vi "UI_GUI.vi"() -> ()   [LabVIEW 2014]
uses:
  <vilib>/addons/database/Connection.llb/DB Tools Open Connec (String).vi
  <vilib>/Utility/file.llb/Read From Spreadsheet File (string).vi
  Terminal-Global-SetValues.vi
  <vilib>/addons/database/_DB Variant To Data/Database Variant To Data.xnode
  <vilib>/addons/database/NI_Database_API.lvlib
panel:
  in  "取消":bool
  in  "选项卡控件":enum32{"选项卡 1", "选项卡 2", "选项卡 3", "选项卡 4"}(tab)
  in  "NEXT_1":bool caption="下一步"
  in  "试验人员姓名":string
  in  "试验名称":string
  out "试验日期":string
  in  "径向加载压力":dbl
  in  "轴向加载压力":dbl
  in  "润滑油温度":dbl
  in  "轴承类型":enum32{"角接触球", "圆柱滚子"}(radio)
  in  "BACK_2":bool caption="上一步"
  in  "NEXT_2":bool caption="下一步"
  in  "供油流量":dbl
  in  "供油润滑油温度":dbl caption="供油润滑油温度T"
  in  "下拉列表":u16(ring) items=["", "模板一", "模板二", "模板三"]
  in  "选择文件":path
  in  "BACK_3":bool caption="上一步"
  in  "NEXT_3":bool caption="下一步"
  in  "载荷谱表格":string[][](table)
  out "载荷谱表格显示":string[][](table) caption="载荷谱表格"
  out "润滑油温度显示":dbl caption="润滑油温度"
  out "轴承类型显示":string caption="轴承类型"
  in  "BACK_4":bool caption="上一步"
  out "试验日期显示":string caption="试验日期"
  out "试验人员姓名显示":string caption="试验人员姓名"
  out "试验名称显示":string caption="试验名称"
  out "径向加载压力显示":dbl caption="径向加载压力"
  out "轴向加载压力显示":dbl caption="轴向加载压力"
  out "供油润滑油温度显示":dbl caption="供油润滑油温度T"
  out "供油流量显示":dbl caption="供油流量"
  in  "ok":bool
  # "轴承测试系统"
  # "试验信息输入"
  # "试验轴承类型"
  # "请选择"
  # "试验轴承润滑单元设定"
  # "预载荷及高压顶起载荷设置"
  # "载荷谱设置"
  # "选择载荷谱模板"
  # "导入载荷谱"
  # "请确认您输入的内容"
  # "试验轴承润滑单元参数"
  # "预载荷及高压顶起载荷设置"
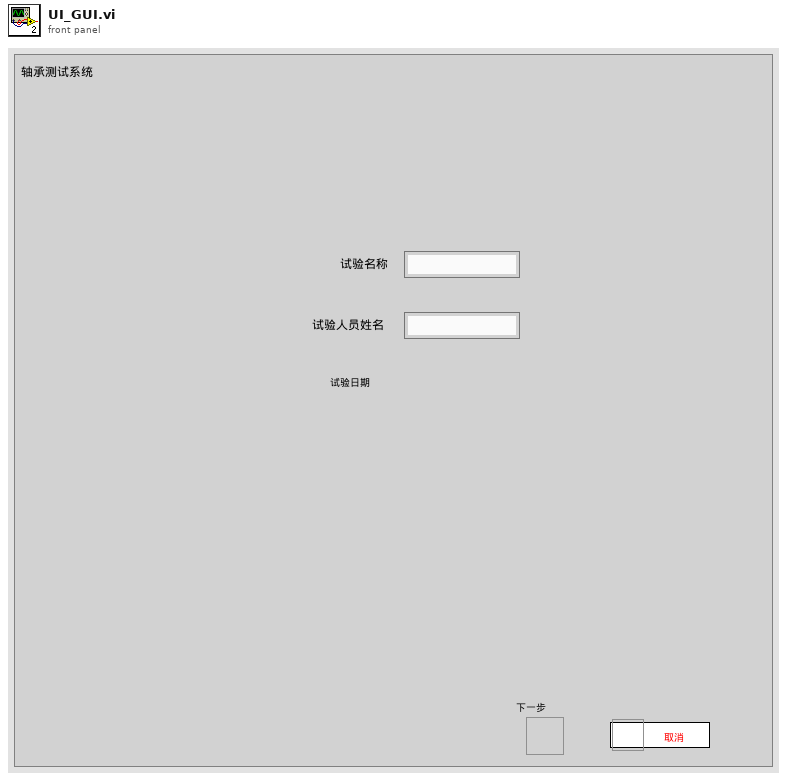
[diagram p1: front panel]
types:
  T1 = enum32{"选项卡 1", "选项卡 2", "选项卡 3", "选项卡 4", "选项卡 5", "选项卡 6", "选项卡 7"}
  T2 = typedef "NI_Database_API.lvlib/Conn ObjectReference.ctl" = refnum<k1>
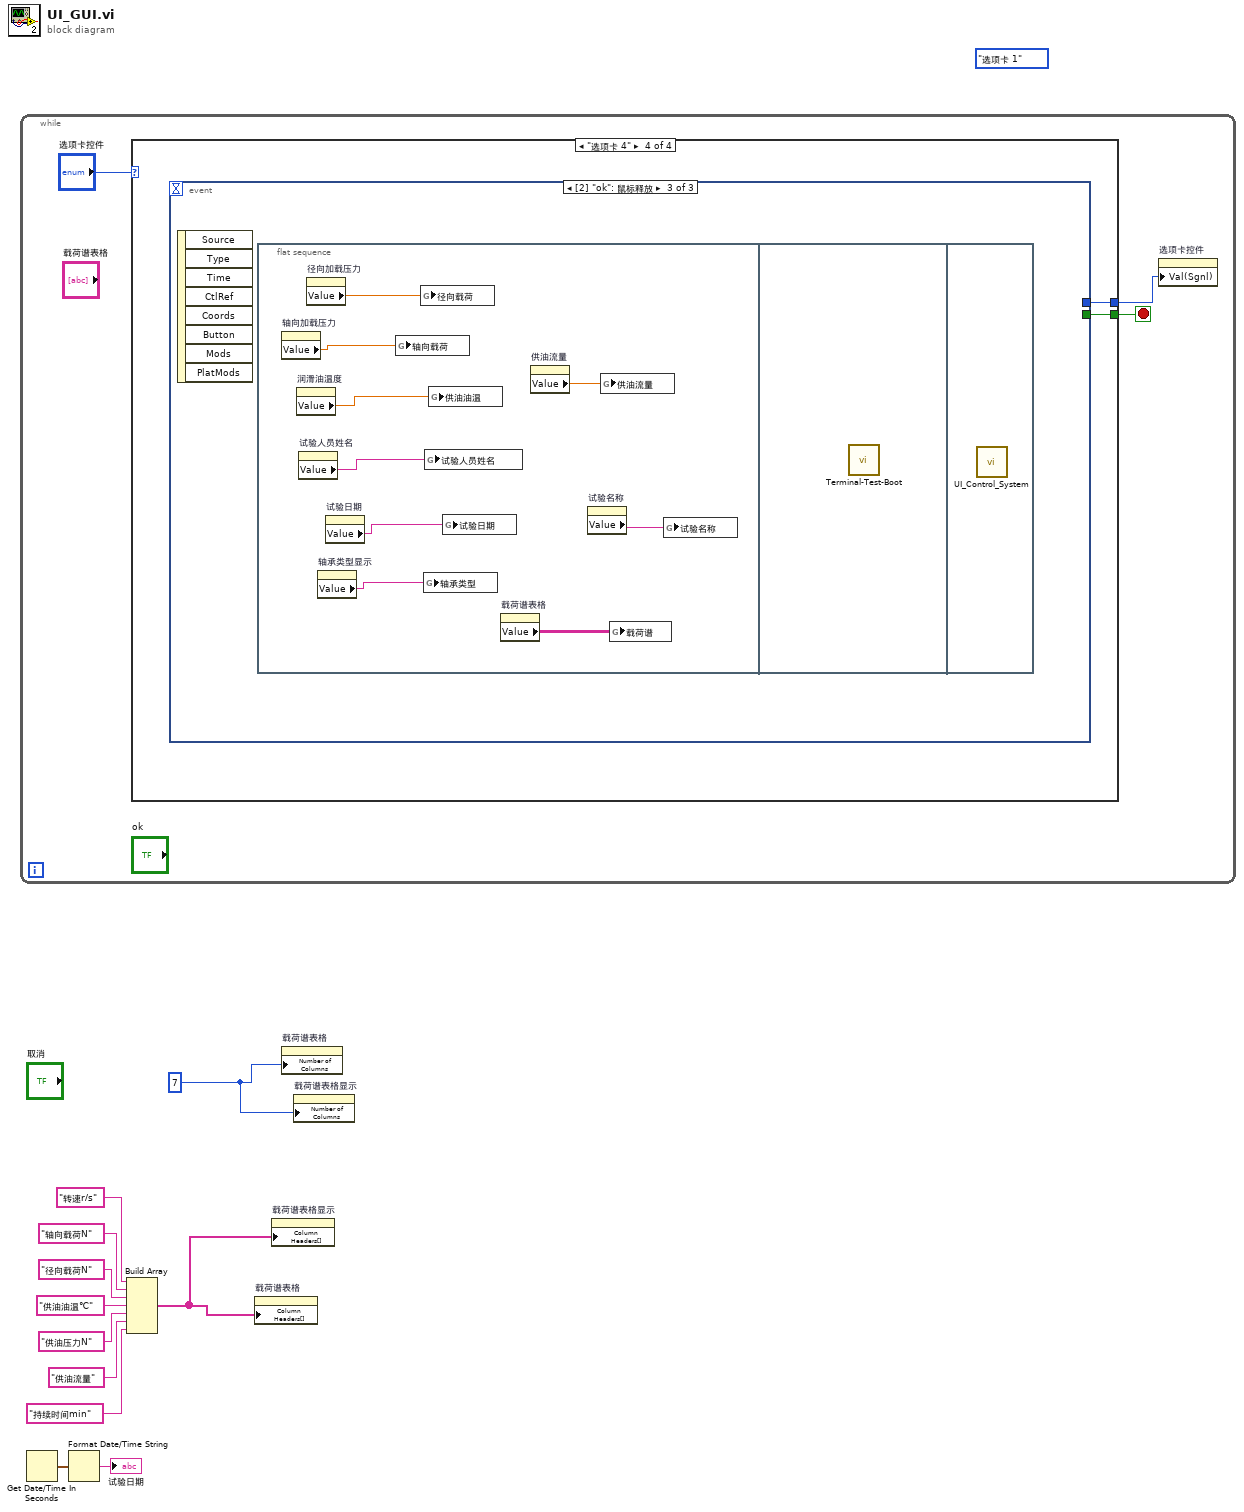
[diagram p0: block diagram]
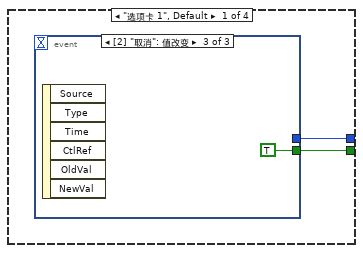
[diagram p2: hidden frame]
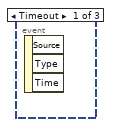
[diagram p3: hidden frame]
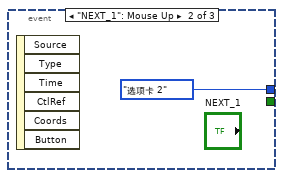
[diagram p4: hidden frame]
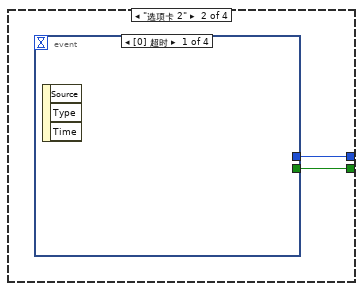
[diagram p5: hidden frame]
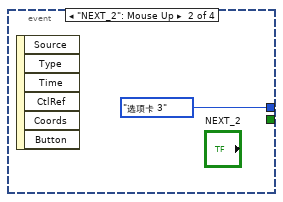
[diagram p6: hidden frame]
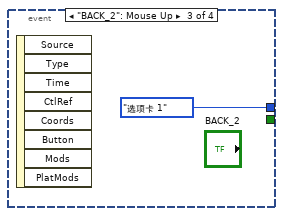
[diagram p7: hidden frame]
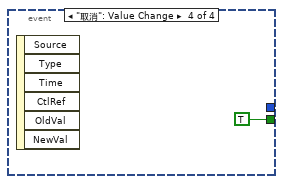
[diagram p8: hidden frame]
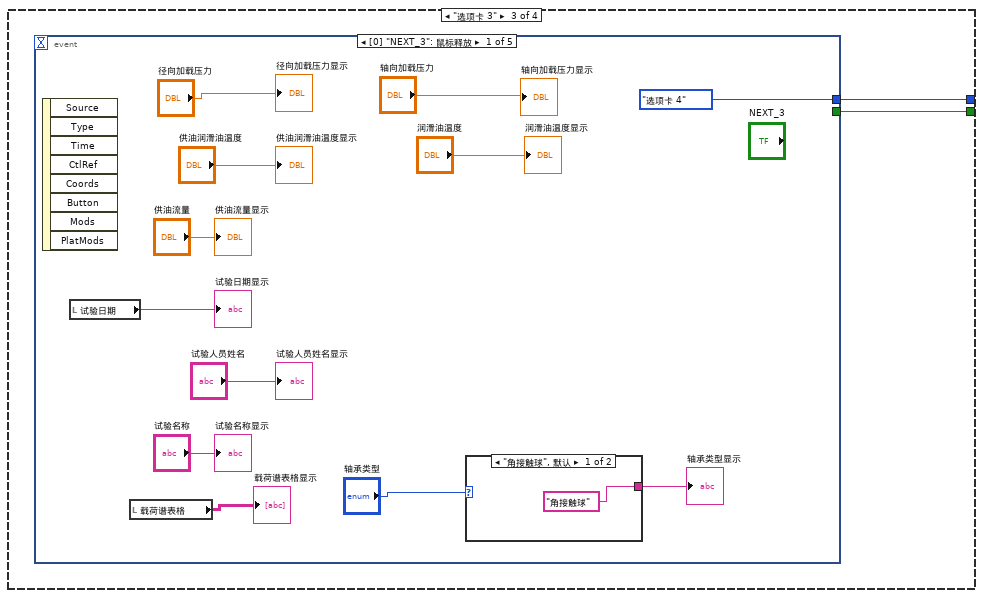
[diagram p9: hidden frame]
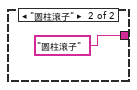
[diagram p10: hidden frame]
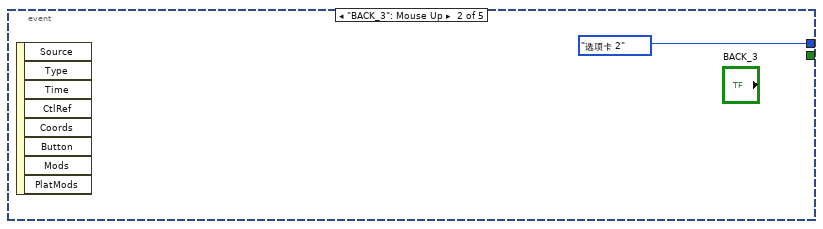
[diagram p11: hidden frame]
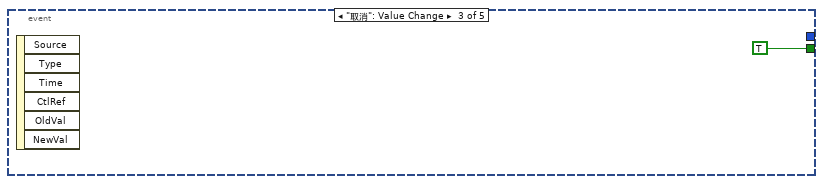
[diagram p12: hidden frame]
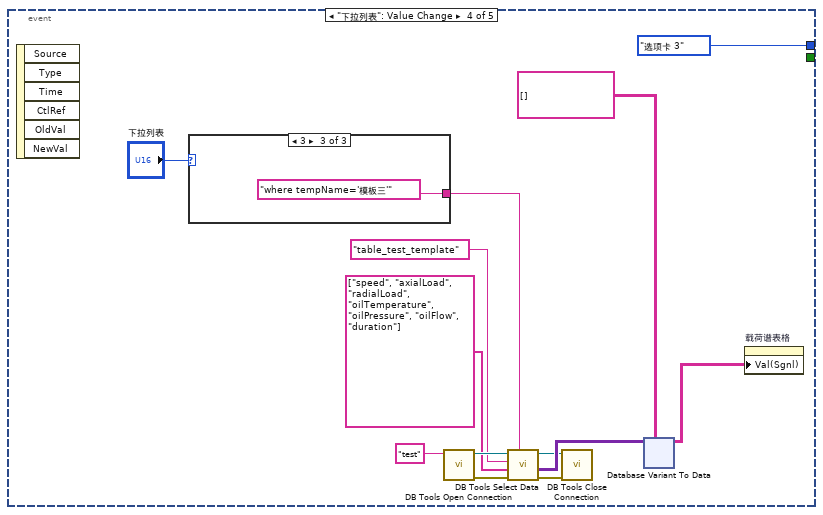
[diagram p13: hidden frame]
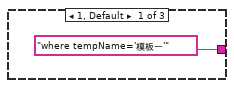
[diagram p14: hidden frame]
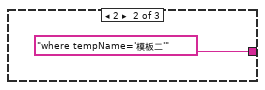
[diagram p15: hidden frame]
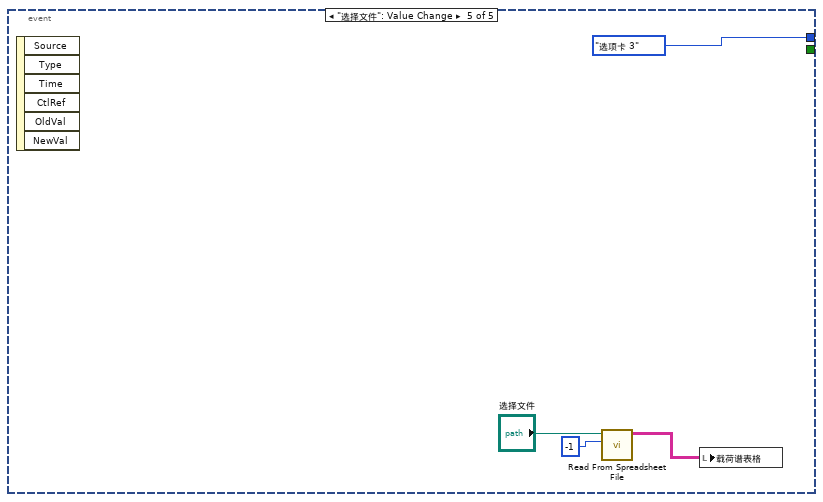
[diagram p16: hidden frame]
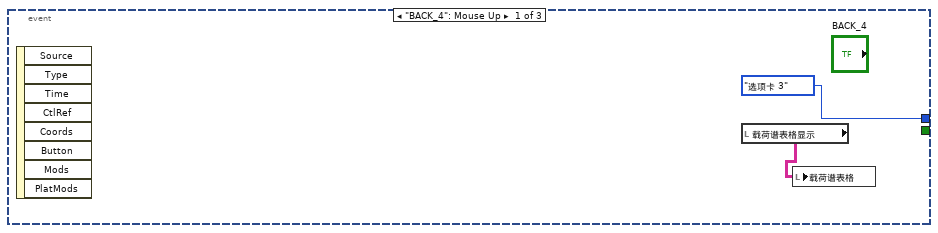
[diagram p17: hidden frame]
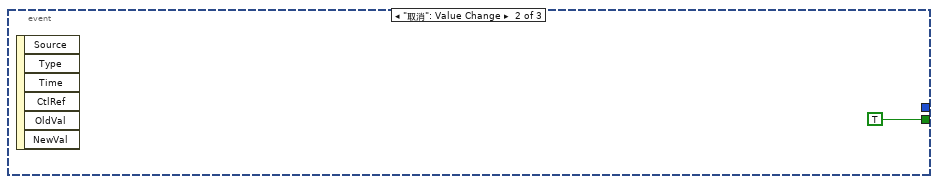
[diagram p18: hidden frame]
diagram:
  w1 = 7
  (unwired) enum32{"选项卡 1", "选项卡 2", "选项卡 3", "选项卡 4"}."选项卡 1" ("选项卡控件")
  n1 = while {
    stop <- w13 stop-if-true
    n2 = case shown="\"选项卡 4\"" "选项卡控件" {
      tunnel: [w16 w20 w25 w107] -> w14
      tunnel: [w15 w19 w24 w106] -> w13
      frame "选项卡 1", Default {
        n3 = event shown="[2] \"取消\": 值改变" {
          selector: _ -> [_ _ _]
          dyn-events: _ -> [_ _ _]
          timeout: _ -> [_ _ _]
          tunnel: [_ T1."选项卡 2" ("选项卡控件") _] -> w16
          tunnel: [_ _ TRUE] -> w15
          event Timeout {
            n4 = event-data() -> ()  [unwired: 1 in, 3 out]
          }
          event "NEXT_1": Mouse Up {
            n5 = event-data() -> ()  [unwired: 1 in, 6 out]
          }
          event "取消": Value Change {
            n6 = event-data() -> ()  [unwired: 1 in, 6 out]
          }
        }
      }
      frame "选项卡 2" {
        n7 = event shown="[0] 超时" {
          selector: _ -> [_ _ _ _]
          dyn-events: _ -> [_ _ _ _]
          timeout: _ -> [_ _ _ _]
          tunnel: [_ T1."选项卡 3" ("选项卡控件") T1."选项卡 1" ("选项卡控件") _] -> w20
          tunnel: [_ _ _ TRUE] -> w19
          event Timeout {
            n8 = event-data() -> ()  [unwired: 1 in, 3 out]
          }
          event "NEXT_2": Mouse Up {
            n9 = event-data() -> ()  [unwired: 1 in, 6 out]
          }
          event "BACK_2": Mouse Up {
            n10 = event-data() -> ()  [unwired: 1 in, 8 out]
          }
          event "取消": Value Change {
            n11 = event-data() -> ()  [unwired: 1 in, 6 out]
          }
        }
      }
      frame "选项卡 3" {
        n12 = event shown="[0] \"NEXT_3\": 鼠标释放" {
          selector: _ -> [_ _ _ _ _]
          dyn-events: _ -> [_ _ _ _ _]
          timeout: _ -> [_ _ _ _ _]
          tunnel: [enum32{"选项卡 1", "选项卡 2", "选项卡 3", "选项卡 4"}."选项卡 4" ("选项卡控件") enum32{"选项卡 1", "选项卡 2", "选项卡 3", "选项卡 4"}."选项卡 2" ("选项卡控件") _ T1."选项卡 3" ("选项卡控件") enum32{"选项卡 1", "选项卡 2", "选项卡 3", "选项卡 4"}."选项卡 3" ("选项卡控件")] -> w25
          tunnel: [_ _ TRUE _ _] -> w24
          event "NEXT_3": Mouse Up {
            n13 = event-data() -> ()  [unwired: 1 in, 8 out]
            n14 = local read "试验日期"() -> (→"试验日期显示":string)
            n15 = local read "载荷谱表格"() -> (→"载荷谱表格显示":string[][])
            n16 = case shown="\"角接触球\", 默认" "轴承类型" {
              tunnel: ["角接触球" "圆柱滚子"] -> w27
              frame "角接触球", Default {
              }
              frame "圆柱滚子" {
              }
            }
            "轴承类型显示" <- w27
            "试验名称显示" <- "试验名称"
            "试验人员姓名显示" <- "试验人员姓名"
            "供油流量显示" <- "供油流量"
            "供油润滑油温度显示" <- "供油润滑油温度"
            "径向加载压力显示" <- "径向加载压力"
            "轴向加载压力显示" <- "轴向加载压力"
            "润滑油温度显示" <- "润滑油温度"
          }
          event "BACK_3": Mouse Up {
            n17 = event-data() -> ()  [unwired: 1 in, 8 out]
          }
          event "取消": Value Change {
            n18 = event-data() -> ()  [unwired: 1 in, 6 out]
          }
          event "下拉列表": Value Change {
            n19 = event-data() -> ()  [unwired: 1 in, 6 out]
            n20 = case shown="3" "下拉列表" {
              tunnel: ["where tempName='模板一'" "where tempName='模板二'" "where tempName='模板三'"] -> w43
              frame 1, Default {
              }
              frame 2 {
              }
              frame 3 {
              }
            }
            n21 = call-poly <vilib>:"DB Tools Open Connection.vi"("connection information"="test") -> ("error out"=w45:errorcluster, "connection reference"=w52:T2)  [unwired: 7 in]
            n22 = call <vilib>:"DB Tools Select Data.vi"("condition"=w43, "error in (no error)"=w45, "columns"=string[] ["speed", "axialLoad", "radialLoad", "oilTemperature", "oilPressure", "oilFlow", "duration"], "table"="table_test_template", "connection reference"=w52) -> ("error out"=w46:errorcluster, "data"=w49:variant[][], "connection reference out"=w47:T2)  [unwired: 1 in]
            n23 = call <vilib>:"DB Tools Close Connection.vi"("error in (no error)"=w46, "connection reference"=w47) -> ()  [unwired: 5 in, 1 out]
            n24 = xnode "Database Variant To Data"("database variant"=w49, "type"=string[][] []) -> ("data"=w42:string[][])  [unwired: 1 in, 1 out]
            n25 = property on="载荷谱表格" class="Tbl (严格)"("Val(Sgnl)"=w42) -> ()  [unwired: 2 in, 2 out]
          }
          event "选择文件": Value Change {
            n26 = event-data() -> ()  [unwired: 1 in, 6 out]
            n27 = call-poly <vilib>:"Read From Spreadsheet File.vi"("number of rows (all:-1)"=-1, "file path (dialog if empty)"="选择文件") -> ("all rows"=w102:string[][])  [unwired: 5 in, 4 out]
            n28 = local write "载荷谱表格"(w102) -> ()
          }
        }
      }
      frame "选项卡 4" {
        n29 = event shown="[2] \"ok\": 鼠标释放" {
          selector: _ -> [_ _ _]
          dyn-events: _ -> [_ _ _]
          timeout: _ -> [_ _ _]
          tunnel: [enum32{"选项卡 1", "选项卡 2", "选项卡 3", "选项卡 4"}."选项卡 3" ("选项卡控件") _ _] -> w107
          tunnel: [_ TRUE _] -> w106
          event "BACK_4": Mouse Up {
            n30 = event-data() -> ()  [unwired: 1 in, 8 out]
            n31 = local read "载荷谱表格显示"() -> (w108:string[][])
            n32 = local write "载荷谱表格"(w108) -> ()
          }
          event "取消": Value Change {
            n33 = event-data() -> ()  [unwired: 1 in, 6 out]
          }
          event "ok": Mouse Up {
            n34 = event-data() -> ()  [unwired: 1 in, 8 out]
            n35 = flat-sequence {
              frame #0 {
                n36 = property on="轴向加载压力" class="DigNum (严格)"() -> ("Value"=w118:dbl)  [unwired: 2 in, 2 out]
                n37 = property on="润滑油温度" class="DigNum (严格)"() -> ("Value"=w117:dbl)  [unwired: 2 in, 2 out]
                n38 = property on="试验人员姓名" class="Str"() -> ("Value"=w116:string)  [unwired: 2 in, 2 out]
                n39 = property on="径向加载压力" class="DigNum (严格)"() -> ("Value"=w119:dbl)  [unwired: 2 in, 2 out]
                n40 = property on="轴承类型显示" class="Str"() -> ("Value"=w114:string)  [unwired: 2 in, 2 out]
                n41 = property on="试验日期" class="Str"() -> ("Value"=w115:string)  [unwired: 2 in, 2 out]
                n42 = global write "Terminal-Global-SetValues.vi" "轴向载荷"(w118) -> ()
                n43 = global write "Terminal-Global-SetValues.vi" "径向载荷"(w119) -> ()
                n44 = global write "Terminal-Global-SetValues.vi" "轴承类型"(w114) -> ()
                n45 = global write "Terminal-Global-SetValues.vi" "试验人员姓名"(w116) -> ()
                n46 = global write "Terminal-Global-SetValues.vi" "供油油温"(w117) -> ()
                n47 = global write "Terminal-Global-SetValues.vi" "试验日期"(w115) -> ()
                n48 = property on="载荷谱表格" class="Tbl (严格)"() -> ("Value"=w111:string[][])  [unwired: 2 in, 2 out]
                n49 = property on="供油流量" class="DigNum (严格)"() -> ("Value"=w113:dbl)  [unwired: 2 in, 2 out]
                n50 = property on="试验名称" class="Str"() -> ("Value"=w112:string)  [unwired: 2 in, 2 out]
                n51 = global write "Terminal-Global-SetValues.vi" "供油流量"(w113) -> ()
                n52 = global write "Terminal-Global-SetValues.vi" "载荷谱"(w111) -> ()
                n53 = global write "Terminal-Global-SetValues.vi" "试验名称"(w112) -> ()
              }
              frame #1 {
                n54 = call "Terminal-Test-Boot.vi"() -> ()  [unwired: 11 in, 1 out]
              }
              frame #2 {
                n55 = call "UI_Control_System.vi"() -> ()  [unwired: 12 in]
              }
            }
          }
        }
      }
    }
    n56 = property on="选项卡控件" class="TabCtl (严格)"("Val(Sgnl)"=w14) -> ()  [unwired: 2 in, 2 out]
  }
  n57 = Get Date/Time In Seconds() -> (seconds since 1Jan1904=w4:timestamp)
  n58 = Format Date/Time String(seconds (now)=w4) -> (date/time string=→"试验日期":string)  [unwired: 2 in]
  n59 = Build Array("转速r/s", "轴向载荷N", "径向载荷N", "供油油温℃", "供油压力N", "供油流量", "持续时间min") -> (w2:string[])
  n60 = property on="载荷谱表格" class="Tbl (严格)"("Column Headers[]"=w2) -> ()  [unwired: 2 in, 2 out]
  n61 = property on="载荷谱表格显示" class="Tbl (严格)"("Column Headers[]"=w2) -> ()  [unwired: 2 in, 2 out]
  n62 = property on="载荷谱表格" class="Tbl (严格)"("Number of Columns"=w1) -> ()  [unwired: 2 in, 2 out]
  n63 = property on="载荷谱表格显示" class="Tbl (严格)"("Number of Columns"=w1) -> ()  [unwired: 2 in, 2 out]
